vi "Init_stim_digital_tasks_NI.vi"(6 "error in":errorcluster, 8 "Run mode":T1, 9 "Device parameters":T2={"Triggered?"=FALSE, "Shutter channel"="", "Acquisition channels"="", "Acquisition sample rate"=0.0, "Read chunk size"=0, "Stimulation channel"="Dev1/ao0", "Stimulation sample rate"=0.0} {"Read chunk size" min=100 max=100000; "Acquisition sample rate" min=10.0 max=10000.0 step=10.0; "Stimulation sample rate" min=10.0 max=10000.0}) -> (0 "error out":errorcluster, 3 "Stim task out":refnum<k21>)   [LabVIEW 2010]
uses:
  typedefs/device_parameters.ctl
  typedefs/run_mode.ctl
  <vilib>/DAQmx/create/channels.llb/DAQmx Create Channel (DO-Digital Output).vi
  <vilib>/DAQmx/configure/timing.llb/DAQmx Timing (Sample Clock).vi
  <vilib>/DAQmx/configure/trigger.llb/DAQmx Start Trigger (Digital Edge).vi
  Program Files/National Instruments/LabVIEW 2010/resource/objmgr/daqmx.rc
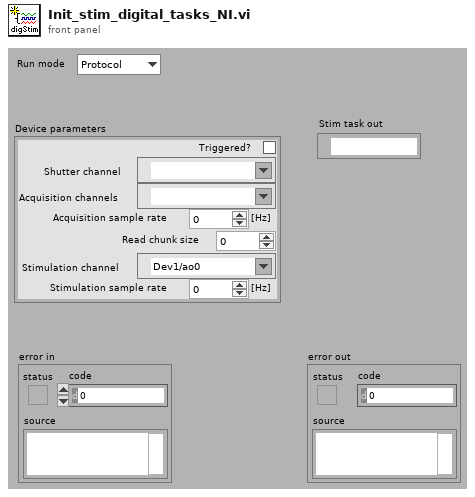
[diagram p1: front panel]
types:
  T1 = typedef "run_mode.ctl" = enum32{"Protocol", "Free Run"}
  T2 = typedef "device_parameters.ctl" = cluster{"Triggered?":bool, "Shutter channel":tag, "Acquisition channels":tag, "Acquisition sample rate":dbl, "Read chunk size":i32, "Stimulation channel":tag, "Stimulation sample rate":dbl}
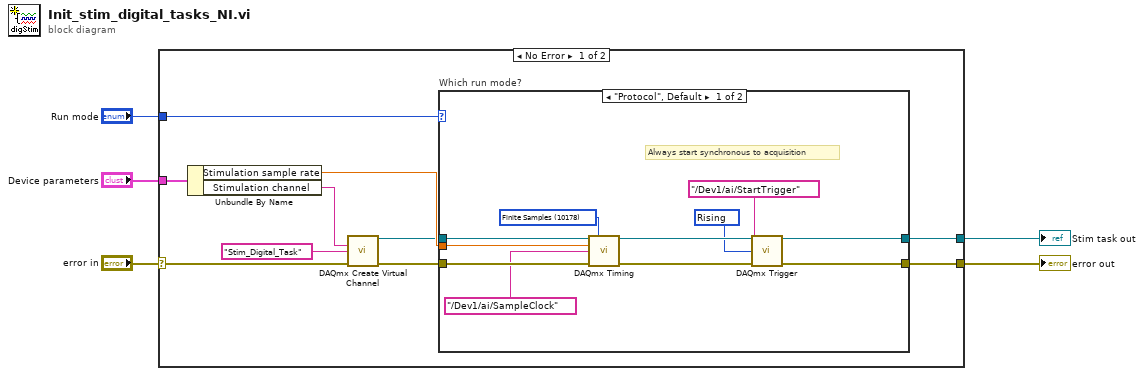
[diagram p0: block diagram]
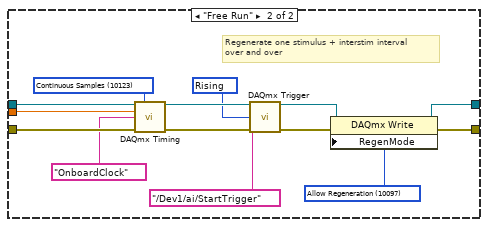
[diagram p2: hidden frame]
diagram:
  n1 = case shown="No Error" "error in" {
    selector: "error in" -> [w8 w41]
    tunnel: [w7 w41] -> w5
    tunnel: "Device parameters" -> [w9 _]
    tunnel: [w10 _] -> w3
    tunnel: "Run mode" -> [w6 _]
    frame No Error {
      n2 = Unbundle By Name(w9) -> ("Stimulation sample rate"=w15:dbl, "Stimulation channel"=w13:tag)
      n3 = call-poly <vilib>:"DAQmx Create Virtual Channel.vi"("lines"=w13, "name to assign"="Stim_Digital_Task", "error in"=w8) -> ("task out"=w11:refnum<k21>, "error out"=w14:errorcluster)  [unwired: 11 in]
      n4 = case "Which run mode?" shown="\"Protocol\", Default" w6 {
        tunnel: w15 -> [w24 w38]
        tunnel: w14 -> [w23 w37]
        tunnel: w11 -> [w22 w36]
        tunnel: [w21 w28] -> w10
        tunnel: [w20 w29] -> w7
        frame "Protocol", Default {
          w16 = 10280 items=["Rising"=10280, "Falling"=10171] ("edge")
          w18 = 10178 items=["Finite Samples"=10178, "Continuous Samples"=10123, "Hardware Timed Single Point"=12522] ("sample mode")
          # "Always start synchronous to acquisition"
          n5 = call-poly <vilib>:"DAQmx Timing.vi"("task/channels in"=w22, "sample mode"=w18, "rate"=w24, "source"=tag "/Dev1/ai/SampleClock", "error in"=w23) -> ("task out"=w26:refnum<k21>, "error out"=w25:errorcluster)  [unwired: 9 in]
          n6 = call-poly <vilib>:"DAQmx Trigger.vi"("task/channels in"=w26, "source"=tag "/Dev1/ai/StartTrigger", "edge"=w16, "error in"=w25) -> ("task out"=w21:refnum<k21>, "error out"=w20:errorcluster)  [unwired: 10 in]
        }
        frame "Free Run" {
          w27 = 10097 items=["Allow Regeneration"=10097, "Do Not Allow Regeneration"=10158] ("RegenMode")
          w32 = 10280 items=["Rising"=10280, "Falling"=10171] ("edge")
          w34 = 10123 items=["Finite Samples"=10178, "Continuous Samples"=10123, "Hardware Timed Single Point"=12522] ("sample mode")
          # "Regenerate one stimulus + interstim interval\nover and over"
          n7 = call-poly <vilib>:"DAQmx Timing.vi"("task/channels in"=w36, "sample mode"=w34, "rate"=w38, "source"=tag "OnboardClock", "error in"=w37) -> ("task out"=w40:refnum<k21>, "error out"=w39:errorcluster)  [unwired: 9 in]
          n8 = call-poly <vilib>:"DAQmx Trigger.vi"("task/channels in"=w40, "source"=tag "/Dev1/ai/StartTrigger", "edge"=w32, "error in"=w39) -> ("task out"=w31:refnum<k21>, "error out"=w30:errorcluster)  [unwired: 10 in]
          n9 = property class="DAQmx Write"(reference=w31, error in=w30, "RegenMode"=w27) -> (reference out=w28:refnum<k21>, error out=w29:errorcluster)
        }
      }
    }
    frame Error {
    }
  }
  "error out" <- w5
  "Stim task out" <- w3
